vi "General Config Test.vi"() -> ()   [LabVIEW 2021]
uses:
  <vilib>/WebDAVClient/NI_WebDAV.lvlib
  <vilib>/WebDAVClient/Advanced/Get Buffer.vi
  Ethernet/Ethernet.lvclass
panel:
  out "Original XML":string
  out "x = y?":bool
  out "LV XML out":string
  out "error out":errorcluster
  in  "IP Address":string
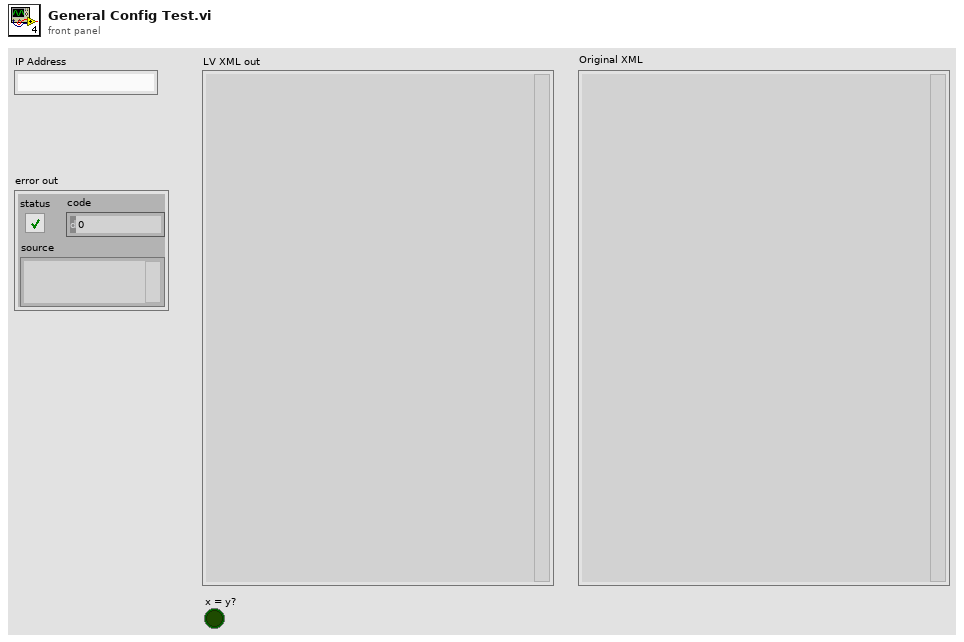
[diagram p1: front panel]
types:
  T1 = typedef "NI_WebDAV.lvlib/SessionHandle.ctl" = refnum<k1>
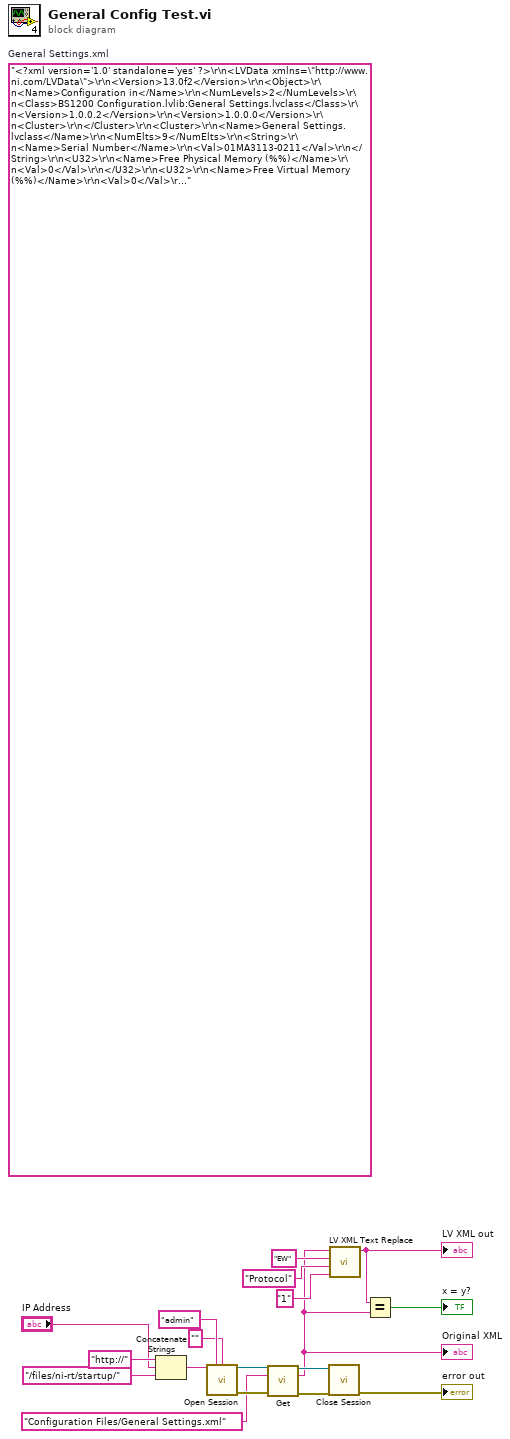
[diagram p0: block diagram]
diagram:
  (unwired) "<?xml version='1.0' standalone='yes' ?>\r\n<LVData xmlns=\"http://www.ni.com/LVData\">\r\n<Version>13.0f2</Version>\r\n<Object>\r\n<Name>Configuration in</Name>\r\n<NumLevels>2</NumLevels>\r\n<Class>BS1200 Configuration.lvlib:General Settings.lvclass</Class>\r\n<Version>1.0.0.2</Version>\r\n<Version>1.0.0.0</Version>\r\n<Cluster>\r\n</Cluster>\r\n<Cluster>\r\n<Name>General Settings.lvclass</Name>\r\n<NumElts>9</NumElts>\r\n<String>\r\n<Name>Serial Number</Name>\r\n<Val>01MA3113-0211</Val>\r\n</String>\r\n<U32>\r\n<Name>Free Physical Memory (%%)</Name>\r\n<Val>0</Val>\r\n</U32>\r\n<U32>\r\n<Name>Free Virtual Memory (%%)</Name>\r\n<Val>0</Val>\r\n</U32>\r\n<String>\r\n<Name>Firmware Revision</Name>\r\n<Val>1.4.0</Val>\r\n</String>\r\n<Timestamp>\r\n<Name>Calibration Date</Name>\r\n<Cluster>\r\n<Name></Name>\r\n<NumElts>4</NumElts>\r\n<I32>\r\n<Name></Name>\r\n<Val>0</Val>\r\n</I32>\r\n<I32>\r\n<Name></Name>\r\n<Val>-816713016</Val>\r\n</I32>\r\n<I32>\r\n<Name></Name>\r\n<Val>-1874952192</Val>\r\n</I32>\r\n<I32>\r\n<Name></Name>\r\n<Val>0</Val>\r\n</I32>\r\n</Cluster>\r\n</Timestamp>\r\n<EW>\r\n<Name>Protocol</Name>\r\n<Choice>CAN</Choice>\r\n<Choice>TCPIP</Choice>\r\n<Val>%d</Val>\r\n</EW>\r\n<Boolean>\r\n<Name>Configured Flag</Name>\r\n<Val>1</Val>\r\n</Boolean>\r\n<Boolean>\r\n<Name>FTP Enabled</Name>\r\n<Val>0</Val>\r\n</Boolean>\r\n<Boolean>\r\n<Name>Aux IO</Name>\r\n<Val>0</Val>\r\n</Boolean>\r\n</Cluster>\r\n</Object>\r\n</LVData>"  # General Settings.xml
  n1 = Concatenate Strings("http://" ("string"), "IP Address", "/files/ni-rt/startup/" ("string")) -> (w16:string)
  n2 = call <vilib>:"Open Session.vi"("host uri prefix"=w16, "username"="admin", "password"="") -> ("session handle out"=w11:T1, "error out"=w12:errorcluster)  [unwired: 11 in]
  n3 = call-poly <vilib>:"Get.vi"("session handle"=w11, "relative uri"="Configuration Files/General Settings.xml" ("string"), "error in (no error)"=w12) -> ("session handle out"=w10:T1, "data"=w1:string, "error out"=w9:errorcluster)  [unwired: 10 in]
  "Original XML" <- w1
  n4 = call <vilib>:"Close Session.vi"("session handle"=w10, "error in (no error)"=w9) -> ("error out"=→"error out":errorcluster)  [unwired: 13 in]
  n5 = call "LV XML Text Replace.vi"("Text"="1", "Tag"="Protocol", "Datatype"="EW", "LV XML in"=w1) -> ("LV XML out"=w3:string)  [unwired: 7 in]
  "LV XML out" <- w3
  n6 = Equal?(x=w3, y=w1) -> (x = y?=→"x = y?":bool)
